vi "DecomposeCovarianceOfPointSetsA&B.vi"(8 "error in (no error)":errorcluster, 11 "Covariance A & B":T1) -> (0 "error out":errorcluster, 3 "R":T1, 4 "Trace(DS)":dbl format="%.2f")   [LabVIEW 2020, in "pointset_utils.lvlib" / "Affine Estimation.lvlib"]
uses:
  Affine Estimation.lvlib
  <vilib>/Analysis/Matrix/Datatypes/RealMatrix.ctl
  <vilib>/Analysis/_algsub.llb/Real Matrix Rank.vi
  <vilib>/Analysis/baseanly.llb/Real A x B.vi
  <vilib>/Analysis/_algsub.llb/Real Matrix Trace.vi
  <vilib>/Analysis/7linalg.llb/SVD Decomposition.vi
  <vilib>/Analysis/7linalg.llb/Real SVD Decomposition.vi
  <vilib>/Analysis/7linalg.llb/Create Special Real Matrix.vi
  <vilib>/Analysis/NI_AALBase.lvlib
  <vilib>/Analysis/NI_AALPro.lvlib
  <vilib>/Analysis/Matrix/NI_Matrix.lvlib
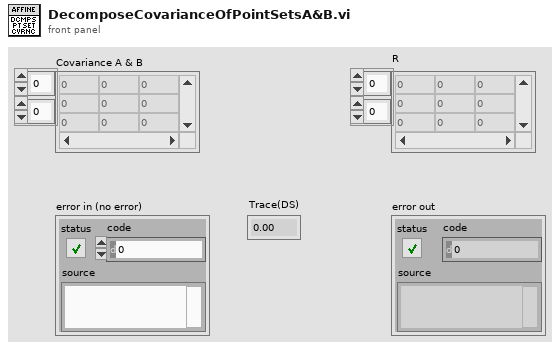
[diagram p1: front panel]
types:
  T1 = typedef "NI_Matrix.lvlib/RealMatrix.ctl" = dbl[][]
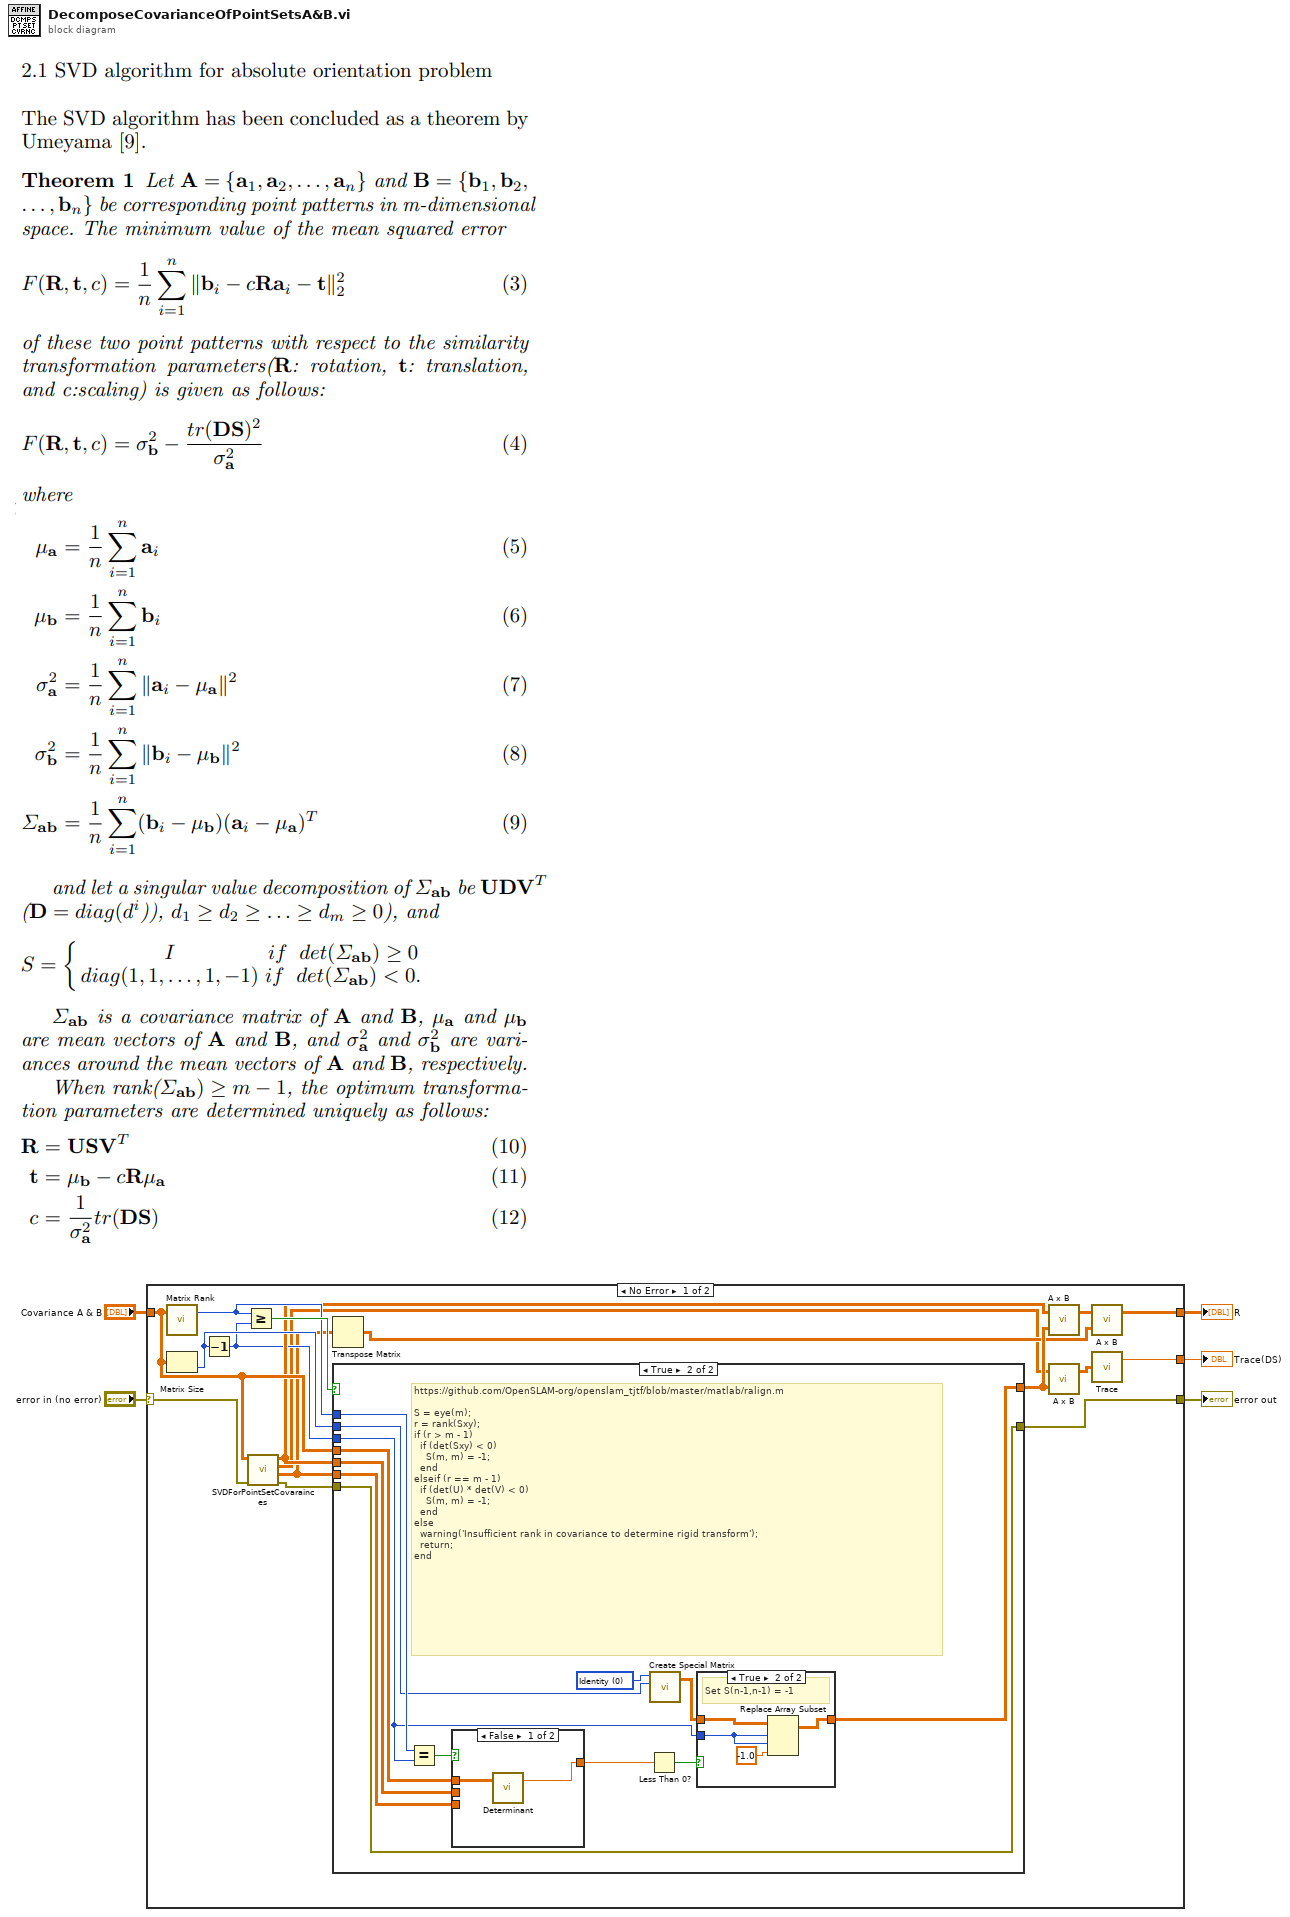
[diagram p0: block diagram]
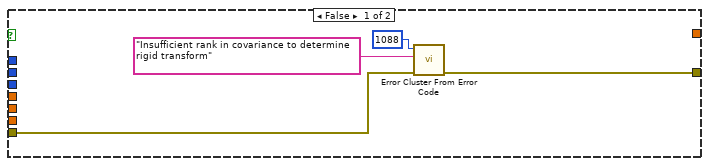
[diagram p2: hidden frame]
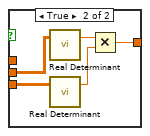
[diagram p4: hidden frame]
diagram:
  n1 = case shown="No Error" "error in (no error)" {
    selector: "error in (no error)" -> [w15 w52]
    tunnel: "Covariance A & B" -> [w18 _]
    tunnel: [w22 w52] -> w4
    tunnel: [w7 _] -> w2
    tunnel: [w6 _] -> w1
    frame No Error {
      n2 = call-poly <vilib>:"Matrix Rank.vi"("Input Matrix"=w18) -> ("rank"=w20:i32)  [unwired: 1 in, 1 out]
      n3 = Matrix Size(0:w18) -> (2:w16:i32)  [unwired: 1 out]
      n4 = Decrement(x=w16) -> (x-1=w10:i32)
      n5 = Greater Or Equal?(x=w20, y=w10) -> (x >= y?=w21:bool)
      n6 = call "SVDForPointSetCovarainces.vi"("error in (no error)"=w15, "Covariance A & B"=w18) -> ("error out"=w14:errorcluster, "V"=w8:T1, "D"=w9:T1, "U"=w11:T1)  [unwired: 6 in]
      n7 = Transpose Matrix(1:w8) -> (0:w12:T1)
      n8 = case shown="True" w21 {
        tunnel: w8 -> [_ w39]
        tunnel: w14 -> [w26 w32]
        tunnel: [w25 w32] -> w22
        tunnel: w16 -> [_ w29]
        tunnel: w20 -> [_ w38]
        tunnel: w18 -> [_ w36]
        tunnel: [_ w33] -> w13
        tunnel: w11 -> [_ w30]
        tunnel: w10 -> [_ w28]
        frame False {
          n9 = call <vilib>:"Error Cluster From Error Code.vi"("error in (no error)"=w26, "error message (\"\")"="Insufficient rank in covariance to determine rigid transform" ("error message (\"\")"), "error code (0)"=1088) -> ("error out"=w25:errorcluster)  [unwired: 6 in]
        }
        frame True {
          w27 = 0 items=["Identity", "Diagonal", "Toeplitz", "Vandermonde", "Companion", "Hankel", "Hadamard", "Wilkinson", "Hilbert", "Inverse Hilbert", "Rosser", "Pascal"] ("matrix type")
          # "https://github.com/OpenSLAM-org/openslam_tjtf/blob/master/matlab/ralign.m\n\nS = eye(m);\nr = rank(Sxy);\nif (r > m - 1) \n  if (det(Sxy) < 0)\n    S(m, m) = -1;\n  end\nelseif (r == m - 1)\n  if (det(U) * det(V) < 0)\n    S(m, m) = -1;\n  end\nelse\n  warning('Insufficient rank in covariance to determine rigid transform');\n  return;\nend"
          n10 = Equal?(x=w38, y=w28) -> (x = y?=w37:bool)
          n11 = case shown="False" w37 {
            tunnel: w39 -> [_ w51]
            tunnel: w36 -> [w46 _]
            tunnel: [w45 w48] -> w35
            tunnel: w30 -> [_ w47]
            frame False {
              n12 = call-poly <vilib>:"Determinant.vi"("Input Matrix"=w46) -> ("determinant"=w45:dbl)  [unwired: 1 in, 1 out]
            }
            frame True {
              n13 = call <vilib>:"Real Determinant.vi"("Input Matrix"=w47) -> ("determinant"=w50:dbl)  [unwired: 1 in, 1 out]
              n14 = call <vilib>:"Real Determinant.vi"("Input Matrix"=w51) -> ("determinant"=w49:dbl)  [unwired: 1 in, 1 out]
              n15 = Multiply(x=w50, y=w49) -> (x*y=w48:dbl)
            }
          }
          n16 = Less Than 0?(x=w35) -> (x < 0?=w34:bool)
          n17 = call-poly <vilib>:"Create Special Matrix.vi"("matrix type"=w27, "matrix size"=w29) -> ("Special Matrix"=w31:T1)  [unwired: 3 in, 1 out]
          n18 = case shown="True" w34 {
            tunnel: w31 -> [w40 w43]
            tunnel: [w40 w42] -> w33
            tunnel: w28 -> [_ w41]
            frame False {
              # "Use S = Identiy Matrix"
            }
            frame True {
              # "Set S(n-1,n-1) = -1"
              n19 = Replace Array Subset(array=w43, new element=-1.0 ("new element/submatrix"), index (row)=w41, index (col)=w41) -> (w42:T1)
            }
          }
        }
      }
      n20 = call-poly <vilib>:"A x B.vi"("B"=w13, "A"=w11) -> ("A x B"=w17:T1)  [unwired: 1 out]
      n21 = call-poly <vilib>:"A x B.vi"("B"=w13, "A"=w9) -> ("A x B"=w19:T1)  [unwired: 1 out]
      n22 = call-poly <vilib>:"A x B.vi"("B"=w12, "A"=w17) -> ("A x B"=w6:T1)  [unwired: 1 out]
      n23 = call-poly <vilib>:"Trace.vi"("Input Matrix"=w19) -> ("trace"=w7:dbl)  [unwired: 1 out]
    }
    frame Error {
    }
  }
  "error out" <- w4
  "Trace(DS)" <- w2
  "R" <- w1
